vi "Black box desired channels.vi"() -> (0 "Names":string[](array[string])=["Range", "Head Gain", "FID(mbar)", "FIDdrive(%)", "Head(C)", "Head(%)", "Fuel(bar)", "Air(bar)", "Exhaust(C)", "Ready?"], 2 "Indicies":i32[](array[numeric])=[14, 19, 23, 24, 27, 28, 31, 32, 33, 41])   [LabVIEW 2022 SP3]
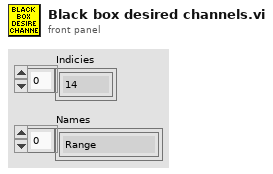
[diagram p1: front panel]
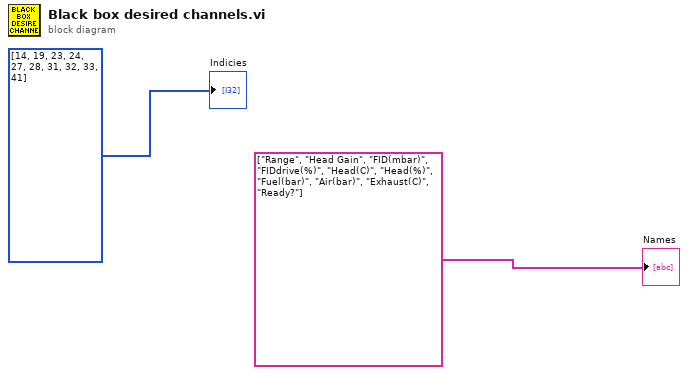
[diagram p0: block diagram]
diagram:
  "Names" <- string[] ["Range", "Head Gain", "FID(mbar)", "FIDdrive(%)", "Head(C)", "Head(%)", "Fuel(bar)", "Air(bar)", "Exhaust(C)", "Ready?"]
  "Indicies" <- i32[] [14, 19, 23, 24, 27, 28, 31, 32, 33, 41]
